vi "Map Controls.vi"(8 "error in":errorcluster, 11 "Instruments in":refnum<class "Instruments.lvclass">) -> (0 "error out":errorcluster, 3 "Instruments out":refnum<class "Instruments.lvclass">)   [LabVIEW 2023, in "Instruments.lvlib" / "Instruments.lvclass"]
uses:
  Library/Instruments.lvclass
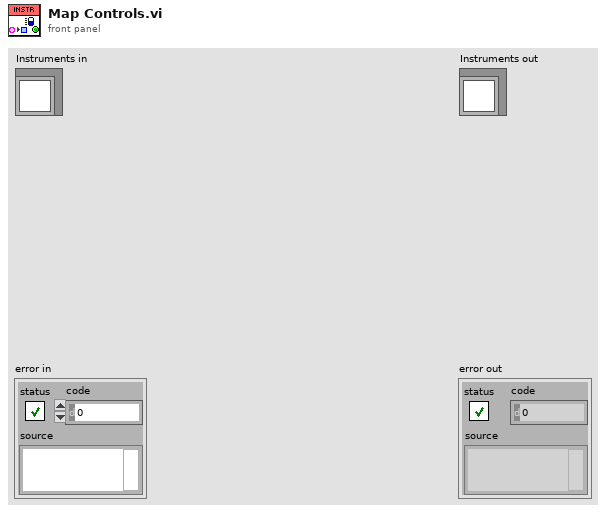
[diagram p1: front panel]
types:
  T1 = typedef "Instruments.lvlib/Instruments.lvclass/Control Element.ctl" = cluster{refnum<vi>, "Label.Text":string}
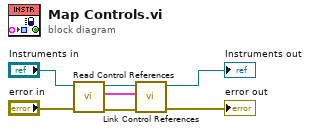
[diagram p0: block diagram]
diagram:
  n1 = call "Read Control References.vi"("error in"="error in", "Instruments in"="Instruments in") -> ("error out"=w3:errorcluster, "Control Map"=w1:T1[], "Instruments out"=w4:refnum<class "Instruments.lvclass">)  [unwired: 7 in]
  n2 = call-dynamic "Link Control References.vi"("error in (no error)"=w3, "Control Map"=w1, "Instruments in"=w4) -> ("error out"=→"error out":errorcluster, "Instruments out"=→"Instruments out":refnum<class "Instruments.lvclass">)  [unwired: 7 in]
